vi "say_hello.vi"(10 "name":string) -> (2 "output":string)   [LabVIEW 2023]
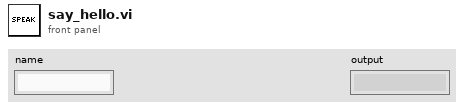
[diagram p1: front panel]
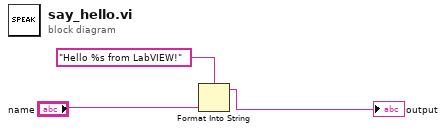
[diagram p0: block diagram]
diagram:
  n1 = Format Into String(format string="Hello %s from LabVIEW!", "name") -> (resulting string=→"output":string)  [unwired: 2 in, 1 out]
